vi "EUI.vi"() -> ()   [LabVIEW 2018]
uses:
  <vilib>/FPGAPlugInAG/cRIO-9034/niLvFpga_Open_cRIO-9034.vi
  <vilib>/rvi/interface/common/dynamic/niFpgaDynamicAddResources.vi
  <vilib>/FPGAPlugInAG/Dynamic/niLvFpga_Reset_Dynamic.vi
  <vilib>/FPGAPlugInAG/Dynamic/niLvFpga_Run_Dynamic.vi
  <vilib>/Utility/error.llb/Error Cluster From Error Code.vi
  <vilib>/rvi/errors/niLvFpgaAdjustHostInterfaceError.vi
  <vilib>/rvi/interface/nirviOpenFPGA/nirviOpenFPGA.xnode
  Bitfiles/NiFpga_VMS_3_Controller.lvbitx
  VMS_3_Controller.vi
  <vilib>/rvi/interface/nirviMethod/nirviMethod.xnode
  <vilib>/rvi/interface/nirviReadWriteControl/nirviReadWriteControl.xnode
  <vilib>/rvi/interface/Simulation/niFpgaSimulationCallBeginRW.vi
  NiFpgaLv.dll
  <vilib>/FPGAPlugInAG/Dynamic/niLvFpga_ReadFifo_Dynamic.vi
  <vilib>/rvi/errors/niLvFpgaMergeErrorWithErrorCode.vi
panel:
  out "FIFO full":bool
  out "last readout error":errorcluster
  in  "Period (ms)":i32=5
  out "error out":errorcluster
  out "Stopped":bool
  in  "Output type":i16=4
  out "Timeouted":bool
  out "Ticks":u64
  out "Ready":bool
  out "Waveform Chart":u32[](graph)
  in  "Operate":bool
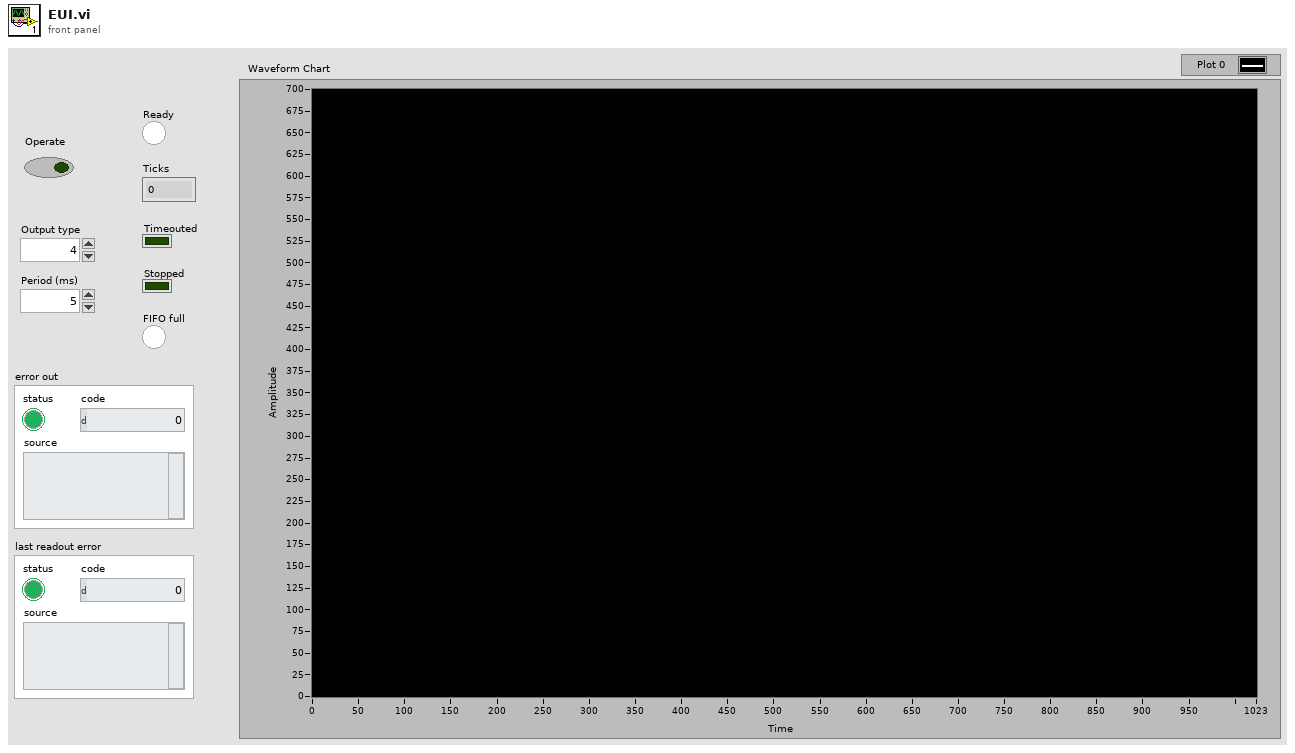
[diagram p1: front panel]
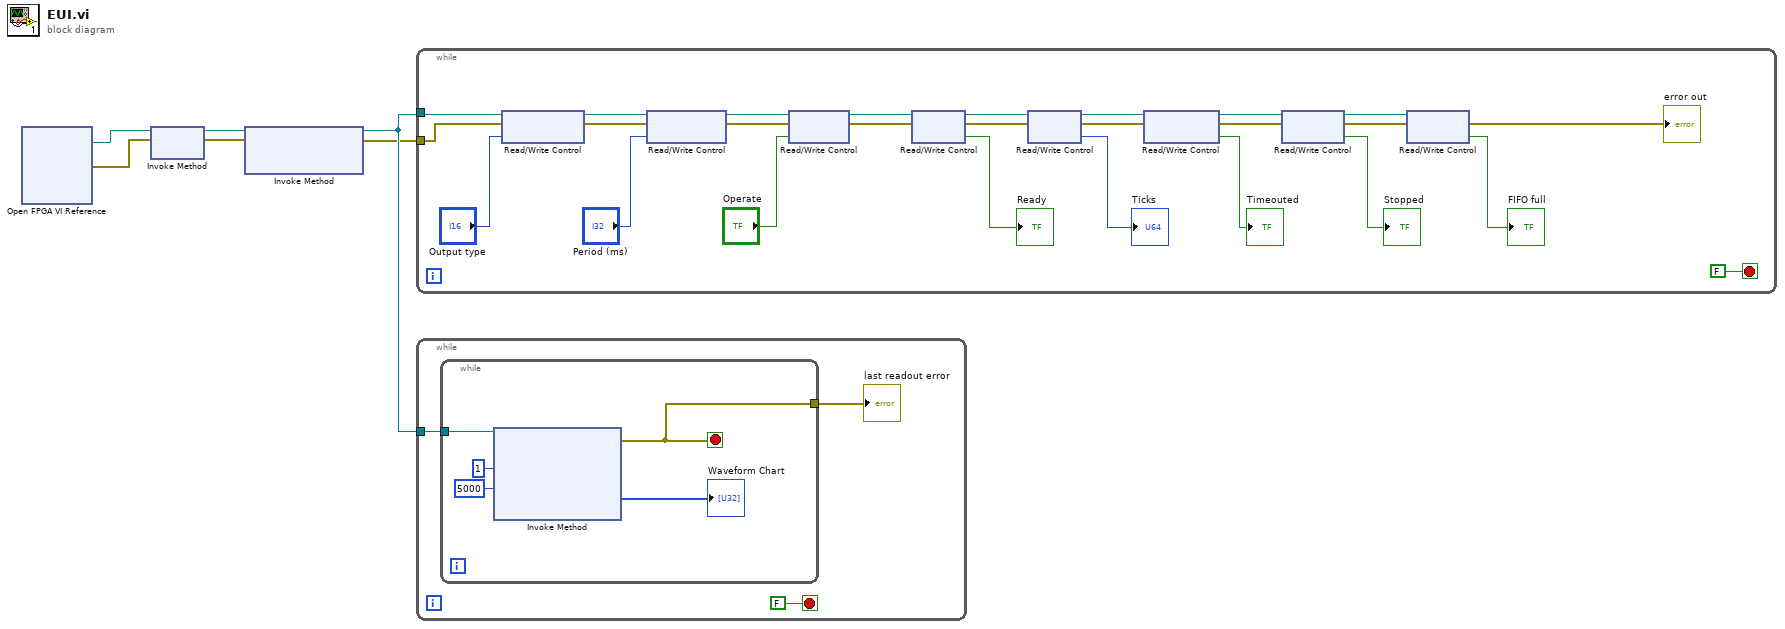
[diagram p0: block diagram]
diagram:
  n1 = xnode "Open FPGA VI Reference"() -> ("FPGA VI Reference Out"=w6:refnum<k20>, "error out"=w2:errorcluster)  [unwired: 2 in]
  n2 = xnode "Invoke Method"("FPGA VI Reference In"=w6, "error in"=w2) -> ("FPGA VI Reference Out"=w3:refnum<k20>, "error out"=w1:errorcluster)
  n3 = xnode "Invoke Method"("FPGA VI Reference In"=w3, "error in"=w1) -> ("FPGA VI Reference Out"=w5:refnum<k20>, "error out"=w4:errorcluster)  [unwired: 1 in]
  n4 = while {
    tunnel: w5 -> [w31]
    tunnel: w4 -> [w19]
    stop <- FALSE stop-if-true
    n5 = xnode "Read/Write Control"("FPGA VI Reference In"=w31, "error in"=w19, "Output type"="Output type") -> ("FPGA VI Reference Out"=w23:refnum<k20>, "error out"=w13:errorcluster)
    n6 = xnode "Read/Write Control"("FPGA VI Reference In"=w23, "error in"=w13, "Period (ms)"="Period (ms)") -> ("FPGA VI Reference Out"=w14:refnum<k20>, "error out"=w12:errorcluster)
    n7 = xnode "Read/Write Control"("FPGA VI Reference In"=w14, "error in"=w12, "Operate"="Operate") -> ("FPGA VI Reference Out"=w29:refnum<k20>, "error out"=w18:errorcluster)
    n8 = xnode "Read/Write Control"("FPGA VI Reference In"=w29, "error in"=w18) -> ("FPGA VI Reference Out"=w27:refnum<k20>, "error out"=w17:errorcluster, "Ready"=→"Ready":bool)
    n9 = xnode "Read/Write Control"("FPGA VI Reference In"=w27, "error in"=w17) -> ("FPGA VI Reference Out"=w25:refnum<k20>, "error out"=w16:errorcluster, "Ticks"=→"Ticks":u64)
    n10 = xnode "Read/Write Control"("FPGA VI Reference In"=w25, "error in"=w16) -> ("FPGA VI Reference Out"=w21:refnum<k20>, "error out"=w15:errorcluster, "Timeouted"=→"Timeouted":bool)
    n11 = xnode "Read/Write Control"("FPGA VI Reference In"=w21, "error in"=w15) -> ("FPGA VI Reference Out"=w8:refnum<k20>, "error out"=w10:errorcluster, "Stopped"=→"Stopped":bool)
    n12 = xnode "Read/Write Control"("FPGA VI Reference In"=w8, "error in"=w10) -> ("error out"=→"error out":errorcluster, "FIFO full"=→"FIFO full":bool)  [unwired: 1 out]
  }
  n13 = while {
    tunnel: w5 -> [w35]
    stop <- FALSE stop-if-true
    n14 = while {
      tunnel: w35 -> [w40]
      tunnel: [w36] -> w33
      stop <- w36 stop-if-true
      n15 = xnode "Invoke Method"("FPGA VI Reference In"=w40, "Number of Elements"=u32 1, "Timeout (ms)"=5000) -> ("error out"=w36:errorcluster, "Data"=→"Waveform Chart":u32[])  [unwired: 1 in, 2 out]
    }
    "last readout error" <- w33
  }
